vi "Image openener.vi"() -> ()   [LabVIEW 2016]
uses:
  <vilib>/vision/NI_Vision_Development_Module.lvlib
panel:
  out "Rectangular spot":T1(plugin-control)
  out "Circle spot":T1(plugin-control)
  in  "size multiplier":i32
  out "Actual ROI":T1(plugin-control)
  out "Parsed array":T1(plugin-control)
  in  "Circle?":bool
  out "ROI Width":i32
  out "ROI Height":i32
  in  "Parse ROI":bool
  in  "Height  step \ndivider":i32=2
  in  "Precision (%)":dbl=90.0 min=1.0 max=100.0 step=1.0 format="%#_3g"
  in  "Spot width":dbl=1.0
  in  "Spot height":dbl=1.0
  in  "EXIT":bool
  out "Opened file  path":path caption="selected path"
  out "Source":T1(plugin-control)
  in  "Open Source":bool
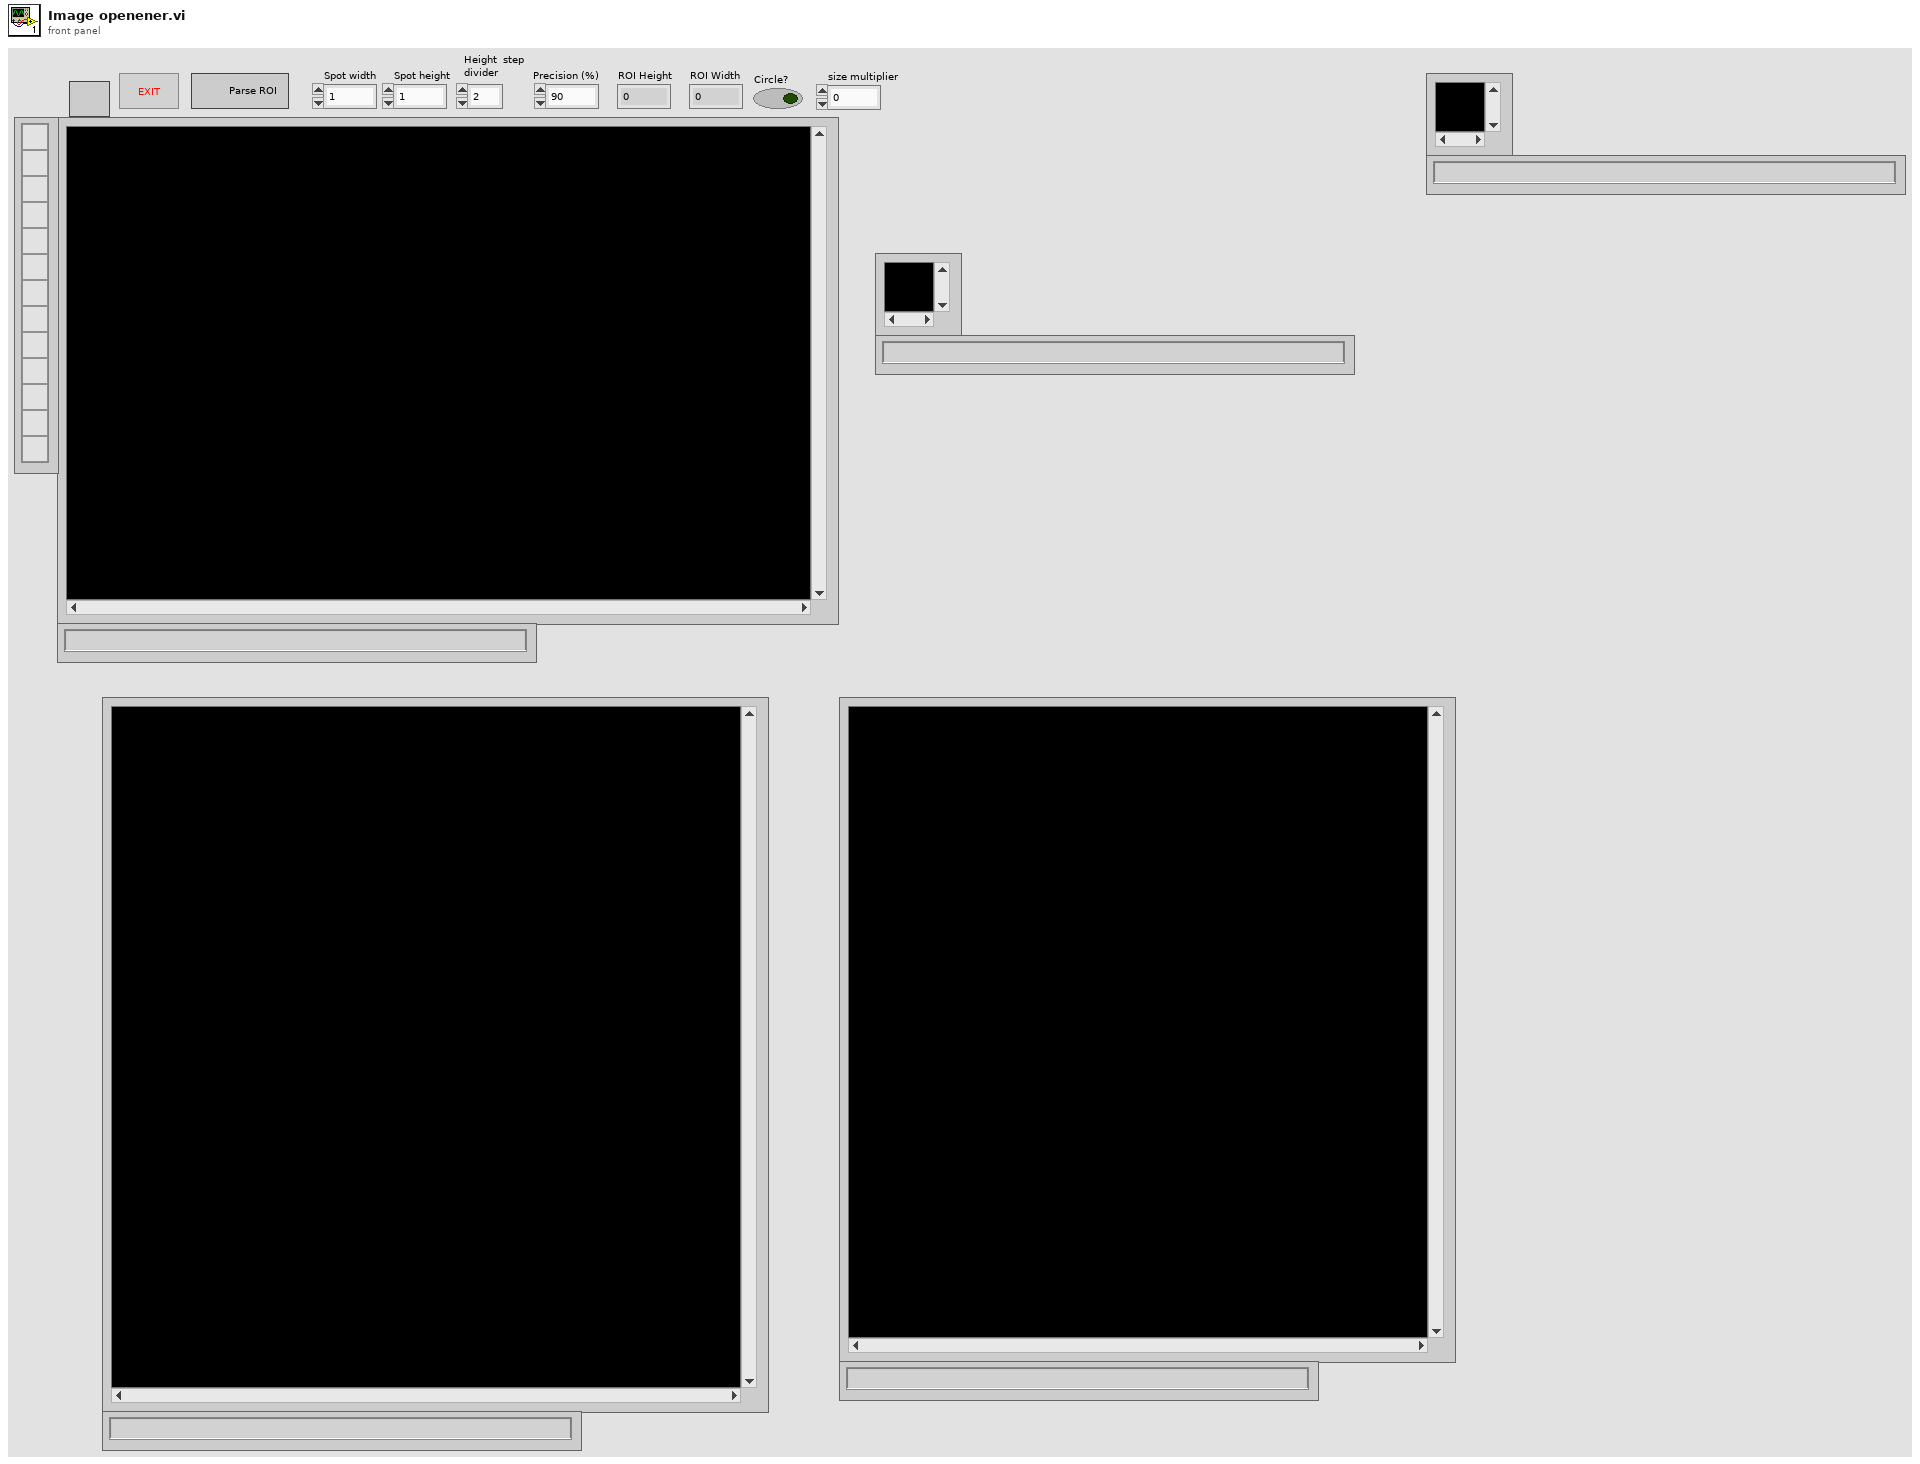
[diagram p1: front panel]
types:
  T1 = typedef "IMAQ Image.ctl" = refnum<image>
  T2 = typedef "Image Type" = u32
  T3 = cluster{"Global Rectangle":i32[], "Contours":cluster{"Contour Type":u32, "ROI Type":u32, "Points":i32[]}[]}
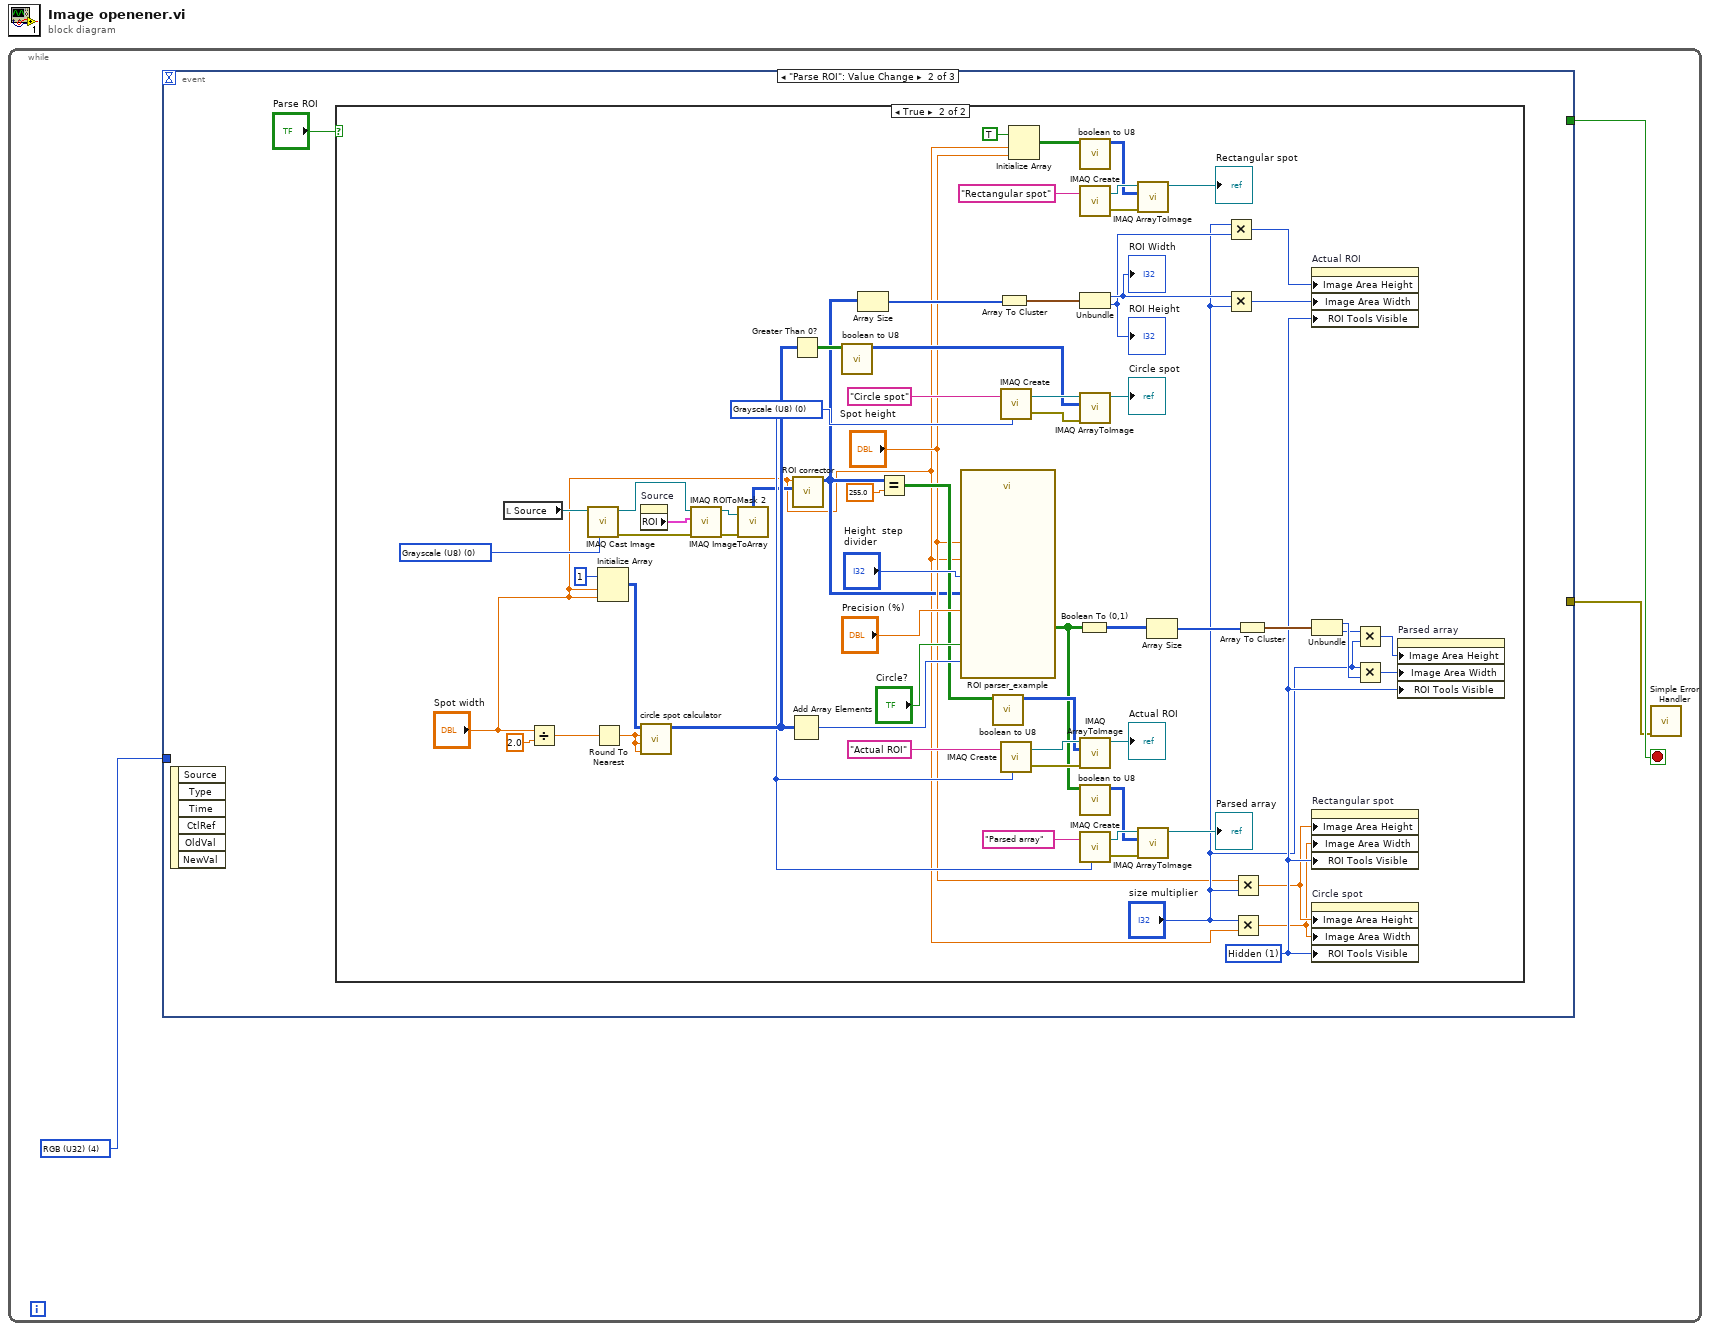
[diagram p0: block diagram]
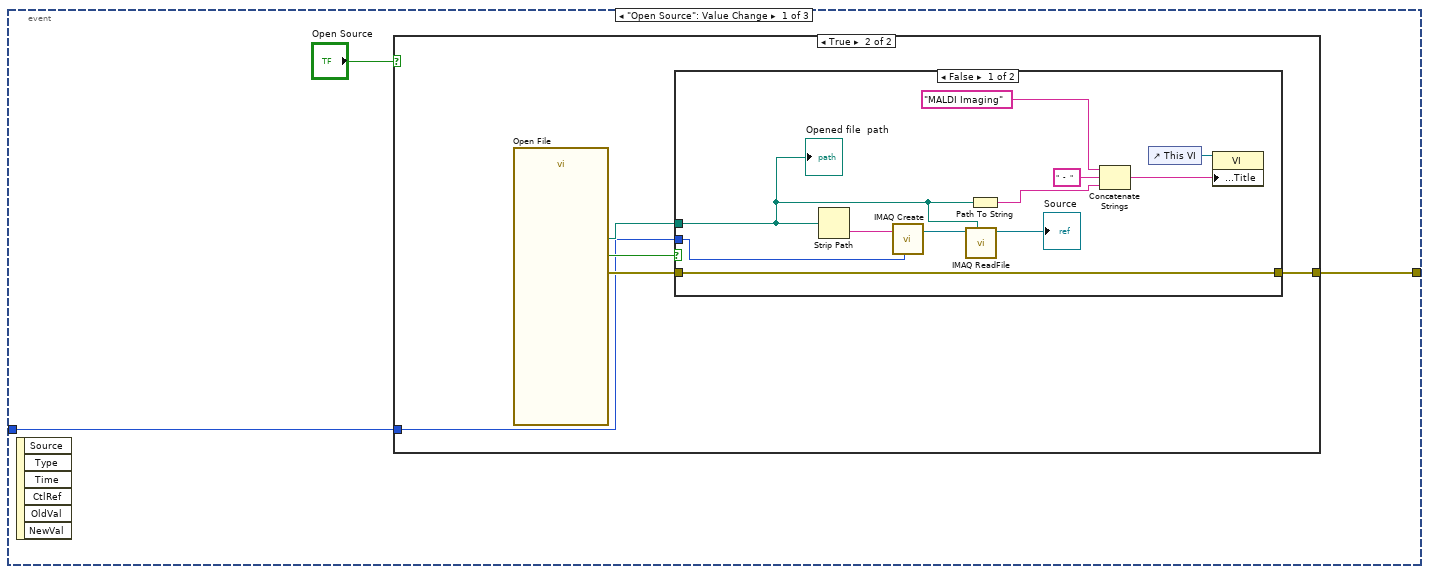
[diagram p2: hidden frame]
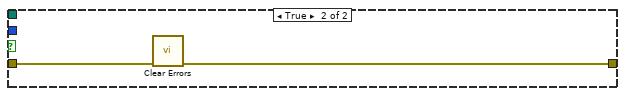
[diagram p4: hidden frame]
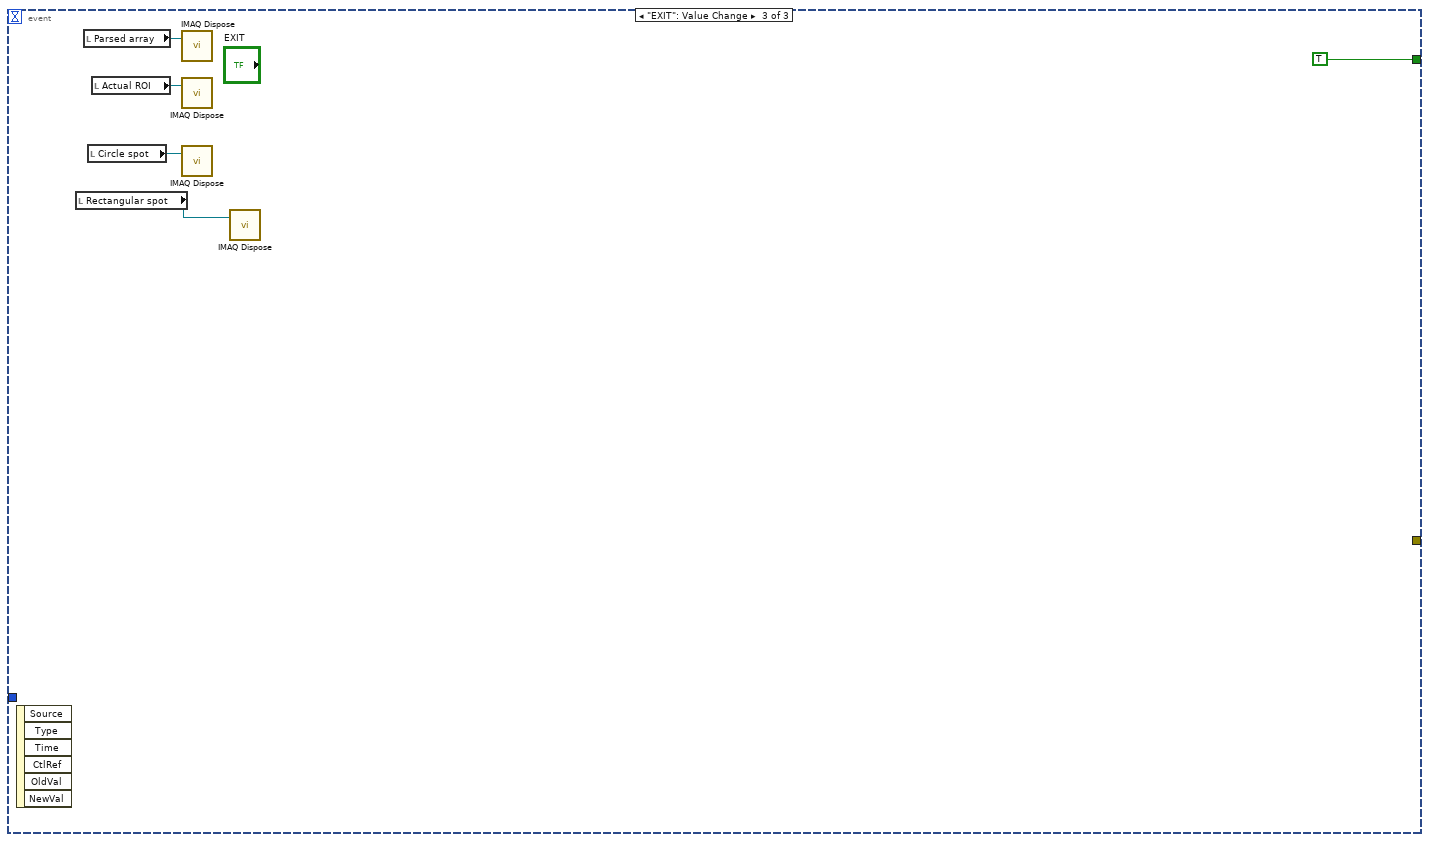
[diagram p6: hidden frame]
diagram:
  n1 = while {
    stop <- w3 stop-if-true
    w2 = T2 4 items=["Grayscale (U8)", "Grayscale (I16)", "Grayscale (SGL)", "Complex (CSG)", "RGB (U32)", "HSL (U32)", "RGB (U64)", "Grayscale (U16)"] ("Image Type")
    n2 = event shown="[1] \"Parse ROI\": Value Change" {
      selector: _ -> [_ _ _]
      dyn-events: _ -> [_ _ _]
      timeout: _ -> [_ _ _]
      tunnel: [_ _ TRUE ("EXIT")] -> w3
      tunnel: w2 -> [w5 _ _]
      tunnel: [w4 _ _] -> w1
      event "Open Source": Value Change {
        n3 = event-data() -> ()  [unwired: 1 in, 6 out]
        n4 = case shown="True" "Open Source" {
          tunnel: w5 -> [_ w8]
          tunnel: [_ w7] -> w4
          frame False {
          }
          frame True {
            n5 = call "Open File"() -> ("selected path"=w11:path, "cancelled"=w9:bool, "error out"=w10:errorcluster)  [unwired: 12 in, 1 out]
            n6 = case shown="False" w9 {
              tunnel: w11 -> [w15 _]
              tunnel: w10 -> [w22 w24]
              tunnel: [w22 w23] -> w7
              tunnel: w8 -> [w12 _]
              frame False {
                n7 = Strip Path(path=w15) -> (name=w14:string)  [unwired: 1 out]
                n8 = call "IMAQ Create"("Image Name"=w14, "Image Type"=w12) -> ("New Image"=w16:T1)  [unwired: 3 in, 1 out]
                n9 = call "IMAQ ReadFile"("File Path"=w15, "Image"=w16) -> ("Image Out"=→"Source":T1)  [unwired: 5 in, 4 out]
                n10 = Path To String(path=w15) -> (string=w19:string)
                n11 = Concatenate Strings("MALDI Imaging" ("string"), "  -  " ("string"), w19) -> (w18:string)
                n12 = control-ref of="This VI"() -> (w17:refnum<vi>)
                n13 = property class="VI"(reference=w17, "Front Panel.Title"=w18) -> ()  [unwired: 1 in, 2 out]
                "Opened file  path" <- w15
              }
              frame True {
                n14 = call <vilib>:"Clear Errors.vi"("error in (no error)"=w24) -> ("error out"=w23:errorcluster)  [unwired: 5 in, 1 out]
              }
            }
          }
        }
      }
      event "Parse ROI": Value Change {
        n15 = event-data() -> ()  [unwired: 1 in, 6 out]
        n16 = case shown="True" "Parse ROI" {
          frame False {
          }
          frame True {
            w34 = u32 1 items=["Visible", "Hidden", "Hidden, Use WindTools Palette"] ("ROI Tools Visible")
            w42 = T2 0 items=["Grayscale (U8)", "Grayscale (I16)", "Grayscale (SGL)", "Complex (CSG)", "RGB (U32)", "HSL (U32)", "RGB (U64)", "Grayscale (U16)"] ("Image Type")
            w88 = T2 0 items=["Grayscale (U8)", "Grayscale (I16)", "Grayscale (SGL)", "Complex (CSG)", "RGB (U32)", "HSL (U32)", "RGB (U64)", "Grayscale (U16)"] ("Image Type")
            n17 = local read "Source"() -> (w90:T1)
            n18 = Divide(x="Spot width", y=2.0) -> (x/y=w75:dbl)
            n19 = call "IMAQ Cast Image"("Image Type"=w88, "Image Src"=w90) -> ("error out"=w87:errorcluster, "Image Dst Out"=w89:T1)  [unwired: 8 in]
            n20 = Round To Nearest(number=w75) -> (nearest integer value=w73:dbl)
            n21 = Initialize Array(1, "Spot width", "Spot width") -> (w76:i32[][])
            n22 = property on="Source" class="ImageControl"() -> ("ROI"=w29:T3)  [unwired: 2 in, 2 out]
            n23 = call "circle spot calculator.vi"("Center Y"=w73, "Radius"=w73, "Center X"=w73, "initialized array"=w76) -> ("Array"=w72:i32[][])  [unwired: 6 in]
            n24 = call "IMAQ ROIToMask 2"("error in (no error)"=w87, "ROI Descriptor"=w29, "Image"=w89) -> ("error out"=w85:errorcluster, "Image Out"=w86:T1)  [unwired: 6 in, 1 out]
            n25 = call "IMAQ ImageToArray"("error in (no error)"=w85, "Image"=w86) -> ("Image Pixels (U8)"=w28:u8[][])  [unwired: 2 in, 4 out]
            n26 = Add Array Elements(numeric array=w72) -> (sum=w71:i32)
            n27 = Greater Than 0?(x=w72) -> (x > 0?=w47:bool[][])
            n28 = call "ROI corrector.vi"("ROI"=w28, "Spot diameter"="Spot width") -> ("Corrected ROI"=w27:u8[][])  [unwired: 9 in]
            n29 = call "boolean to U8.vi"("Boolean array in"=w47) -> ("Array out"=w41:i32[][])  [unwired: 10 in]
            n30 = Array Size(array=w27) -> (size(s)=w81:i32[])
            n31 = Equal?(x=w27, y=255.0) -> (x = y?=w50:bool[][])
            n32 = call "ROI parser_example.vi"("Circle spot"=w71, "Circle?"="Circle?", "ROI (8 bit image)"=w27, "Ablation spot width"="Spot width", "Sampling\nPrecision"="Precision (%)", "Ablation spot heigth"="Spot height", "Height  step \ndivider"="Height  step \ndivider") -> ("Parsed array"=w49:bool[][])  [unwired: 4 in]
            n33 = call "boolean to U8.vi"("Boolean array in"=w50) -> ("Array out"=w56:i32[][])  [unwired: 10 in]
            n34 = Array To Cluster(array=w81) -> (cluster=w82:cluster{"[0]":i32, "[1]":i32})
            n35 = call "IMAQ Create"("Image Name"="Circle spot", "Image Type"=w42) -> ("New Image"=w45:T1, "error out"=w46:errorcluster)  [unwired: 3 in]
            n36 = call "IMAQ Create"("Image Name"="Actual ROI", "Image Type"=w42) -> ("New Image"=w66:T1, "error out"=w67:errorcluster)  [unwired: 3 in]
            n37 = Initialize Array(TRUE, "Spot width", "Spot height") -> (w36:bool[][])
            n38 = Boolean To (0,1)(Boolean=w49) -> (0, 1=w51:i16[][])
            n39 = call "boolean to U8.vi"("Boolean array in"=w36) -> ("Array out"=w35:i32[][])  [unwired: 10 in]
            n40 = call "IMAQ Create"("Image Name"="Rectangular spot") -> ("New Image"=w39:T1, "error out"=w40:errorcluster)  [unwired: 4 in]
            n41 = Unbundle(w82) -> ("[0]"=w62:i32, "[1]"=w61:i32)
            "ROI Height" <- w61
            "ROI Width" <- w62
            n42 = call "IMAQ ArrayToImage"("error in (no error)"=w46, "Image Pixels (U8)"=w41, "Image"=w45) -> ("Image Out"=→"Circle spot":T1)  [unwired: 7 in, 1 out]
            n43 = call "IMAQ ArrayToImage"("error in (no error)"=w67, "Image Pixels (U8)"=w56, "Image"=w66) -> ("Image Out"=→"Actual ROI":T1)  [unwired: 7 in, 1 out]
            n44 = call "boolean to U8.vi"("Boolean array in"=w49) -> ("Array out"=w48:i32[][])  [unwired: 10 in]
            n45 = call "IMAQ Create"("Image Name"="Parsed array", "Image Type"=w42) -> ("New Image"=w69:T1, "error out"=w68:errorcluster)  [unwired: 3 in]
            n46 = call "IMAQ ArrayToImage"("error in (no error)"=w40, "Image Pixels (U8)"=w35, "Image"=w39) -> ("Image Out"=→"Rectangular spot":T1)  [unwired: 7 in, 1 out]
            n47 = call "IMAQ ArrayToImage"("error in (no error)"=w68, "Image Pixels (U8)"=w48, "Image"=w69) -> ("Image Out"=→"Parsed array":T1)  [unwired: 7 in, 1 out]
            n48 = Array Size(array=w51) -> (size(s)=w57:i32[])
            n49 = Multiply(x="size multiplier", y=w61) -> (x*y=w60:i32)
            n50 = Multiply(x=w62, y="size multiplier") -> (x*y=w59:i32)
            n51 = Multiply(x="Spot height", y="size multiplier") -> (x*y=w32:dbl)
            n52 = Multiply(x="size multiplier", y="Spot width") -> (x*y=w31:dbl)
            n53 = Array To Cluster(array=w57) -> (cluster=w58:cluster{"[0]":i32, "[1]":i32})
            n54 = property on="Actual ROI" class="ImageControl"("Image Area Height"=w60, "Image Area Width"=w59, "ROI Tools Visible"=w34) -> ()  [unwired: 2 in, 2 out]
            n55 = Unbundle(w58) -> ("[0]"=w55:i32, "[1]"=w52:i32)
            n56 = property on="Rectangular spot" class="ImageControl"("Image Area Height"=w32, "Image Area Width"=w31, "ROI Tools Visible"=w34) -> ()  [unwired: 2 in, 2 out]
            n57 = property on="Circle spot" class="ImageControl"("Image Area Height"=w32, "Image Area Width"=w31, "ROI Tools Visible"=w34) -> ()  [unwired: 2 in, 2 out]
            n58 = Multiply(x=w52, y="size multiplier") -> (x*y=w53:i32)
            n59 = Multiply(x="size multiplier", y=w55) -> (x*y=w54:i32)
            n60 = property on="Parsed array" class="ImageControl"("Image Area Height"=w53, "Image Area Width"=w54, "ROI Tools Visible"=w34) -> ()  [unwired: 2 in, 2 out]
          }
        }
      }
      event "EXIT": Value Change {
        n61 = event-data() -> ()  [unwired: 1 in, 6 out]
        n62 = local read "Rectangular spot"() -> (w91:T1)
        n63 = local read "Parsed array"() -> (w93:T1)
        n64 = local read "Circle spot"() -> (w92:T1)
        n65 = local read "Actual ROI"() -> (w94:T1)
        n66 = call "IMAQ Dispose"("Image"=w93) -> ()  [unwired: 5 in, 1 out]
        n67 = call "IMAQ Dispose"("Image"=w94) -> ()  [unwired: 5 in, 1 out]
        n68 = call "IMAQ Dispose"("Image"=w92) -> ()  [unwired: 5 in, 1 out]
        n69 = call "IMAQ Dispose"("Image"=w91) -> ()  [unwired: 5 in, 1 out]
      }
    }
    n70 = call <vilib>:"Simple Error Handler.vi"("error in (no error)"=w1) -> ()  [unwired: 4 in, 5 out]
  }
